vi "Write Frequency (kHz).vi"(8 "error in (no error)":errorcluster, 10 "Frequency (Hz)":dbl, 11 "Tone in":refnum<class "Tone.lvclass">) -> (0 "error out":errorcluster, 3 "Tone out":refnum<class "Tone.lvclass">)   [LabVIEW 2020, in "Tone.lvclass"]
uses:
  Tone.lvclass
  Tone.lvclass/Tone.ctl
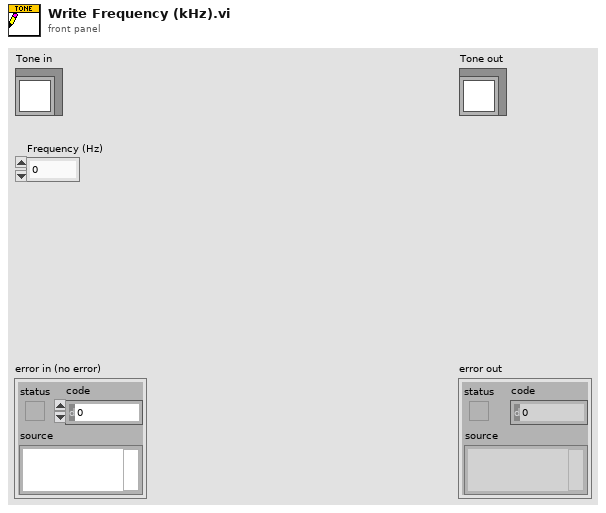
[diagram p1: front panel]
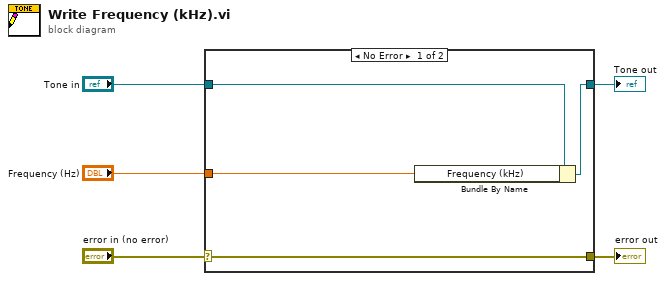
[diagram p0: block diagram]
diagram:
  n1 = case shown="No Error" "error in (no error)" {
    selector: "error in (no error)" -> [w9 w10]
    tunnel: [w9 w10] -> w4
    tunnel: [w7 w11] -> w2
    tunnel: "Tone in" -> [w8 w11]
    tunnel: "Frequency (Hz)" -> [w6 _]
    frame No Error {
      n2 = Bundle By Name(cluster=w8, "Frequency (kHz)"=w6) -> (w7:refnum<class "Tone.lvclass">)
    }
    frame Error {
    }
  }
  "error out" <- w4
  "Tone out" <- w2
